vi "delete element.vi"(8 "program":T1[](array[typedef]) {"n" min=1}, 10 "Del program":bool, 11 "index value":u32[](array[numeric])) -> (0 "program out":T1[](array[typedef]) {"n" min=1})   [LabVIEW 2010]
uses:
  AO n wave.ctl
panel:
  in  "Input Element 2":cluster{"n":i32, "on/off":bool[]}={"n"=1, "on/off"=[FALSE, FALSE, FALSE, FALSE, FALSE, FALSE]}
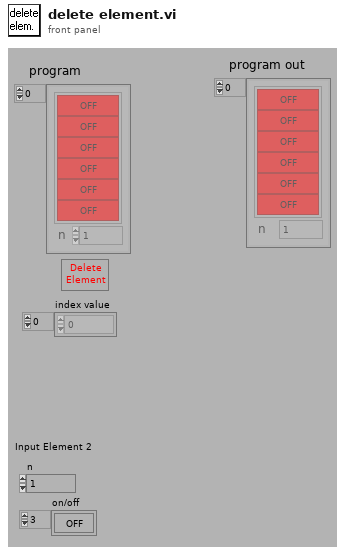
[diagram p1: front panel]
types:
  T1 = typedef "AO n wave.ctl" = cluster{"n":i32, "on/off":bool[]}
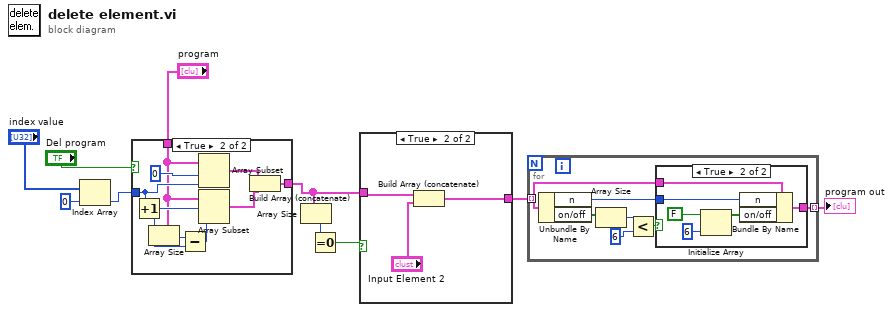
[diagram p0: block diagram]
diagram:
  n1 = Index Array(array="index value", index=0 ("Index")) -> (element=w8:u32)
  n2 = case shown="True" "Del program" {
    tunnel: w8 -> [_ w18]
    tunnel: "program" -> [w11 w17]
    tunnel: [w11 w12] -> w1
    frame False {
    }
    frame True {
      n3 = Increment(x=w18) -> (x+1=w19:u32)
      n4 = Array Size(array=w17) -> (size(s)=w16:i32)
      n5 = Subtract(x=w16, y=w19) -> (x-y=w15:u32)
      n6 = Array Subset(array=w17, index=0 ("Array Index"), length=w18) -> (w13:T1[])
      n7 = Array Subset(array=w17, index=w19, length=w15) -> (w14:T1[])
      n8 = Build Array (concatenate)(w13, w14) -> (w12:T1[])
    }
  }
  n9 = Array Size(array=w1) -> (size(s)=w4:i32)
  n10 = Equal To 0?(x=w4) -> (x = 0?=w3:bool)
  n11 = case shown="True" w3 {
    tunnel: [w21 w23] -> w2
    tunnel: w1 -> [w21 w24]
    frame False {
    }
    frame True {
      n12 = Build Array (concatenate)(w24, "Input Element 2") -> (w23:T1[])
    }
  }
  n13 = for {
    tunnel: w2 -> [w26] mode=indexing
    tunnel: [w25] -> w5 mode=indexing
    n14 = Unbundle By Name(w26) -> ("n"=w27:i32, "on/off"=w28:bool[])
    n15 = Array Size(array=w28) -> (size(s)=w30:i32)
    n16 = Less?(x=w30, y=6) -> (x < y?=w31:bool)
    n17 = case shown="True" w31 {
      tunnel: w27 -> [_ w35]
      tunnel: w26 -> [w32 w34]
      tunnel: [w32 w33] -> w25
      frame False {
      }
      frame True {
        n18 = Initialize Array(FALSE ("channel status"), 6) -> (w36:bool[])
        n19 = Bundle By Name(cluster=w34, "n"=w35, "on/off"=w36) -> (w33:T1)
      }
    }
  }
  "program out" <- w5
